vi "OP600ZP_Softs.vi"(8 "errin":errorcluster caption="entrée d'erreur (pas d'erreur)") -> (0 "errout":errorcluster caption="error out", 3 "OUI/NON":bool)   [LabVIEW 2020]
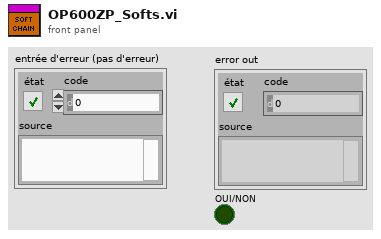
[diagram p1: front panel]
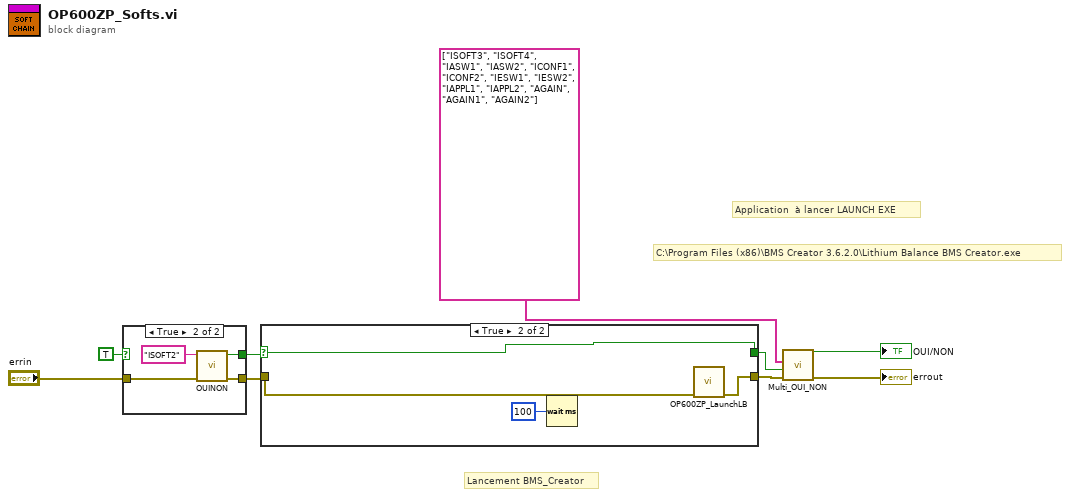
[diagram p0: block diagram]
diagram:
  # "Application  à lancer LAUNCH EXE"
  # "C:\\Program Files (x86)\\BMS Creator 3.6.2.0\\Lithium Balance BMS Creator.exe"
  # "Lancement BMS_Creator"
  n1 = case shown="True" TRUE {
    selector: TRUE -> [w10 _]
    tunnel: "errin" -> [w11 w15]
    tunnel: [w10 w14] -> w9
    tunnel: [w11 w13] -> w8
    frame False {
    }
    frame True {
      n2 = call "OUINON.vi"("errin"=w15, "image"="ISOFT2") -> ("error out"=w13:errorcluster, "OUI/NON"=w14:bool)  [unwired: 8 in]
    }
  }
  n3 = case shown="True" w9 {
    selector: w9 -> [w16 w18]
    tunnel: w8 -> [w17 w21]
    tunnel: [w17 w20] -> w4
    tunnel: [w16 w18] -> w3
    frame False {
    }
    frame True {
      n4 = Wait (ms)(milliseconds to wait=u32 100 ("attente (ms)")) -> ()  [unwired: 1 out]
      n5 = call "OP600ZP_LaunchLB.vi"("errin"=w21) -> ("error out"=w20:errorcluster)  [unwired: 8 in]
    }
  }
  n6 = call "Multi_OUI_NON.vi"("errin"=w4, "errinb"=w3, "Tableau"=string[] ["ISOFT3", "ISOFT4", "IASW1", "IASW2", "ICONF1", "ICONF2", "IESW1", "IESW2", "IAPPL1", "IAPPL2", "AGAIN", "AGAIN1", "AGAIN2"]) -> ("errout"=→"errout":errorcluster, "isok?"=→"OUI/NON":bool)  [unwired: 7 in]
